vi "Select_Filename_List.vi"(4 "No dialogs":bool, 5 "File Type":string, 6 "Search String":string, 7 "At Dialog Prompt Post Process":T1, 8 "Previous Choice":path) -> (0 "Current Results filenames":path[](array[path]), 1 "Selected files":path[](array[path]), 3 "Choosen path":path)   [LabVIEW 2021]
uses:
  Controls/File_Selector_Type.ctl
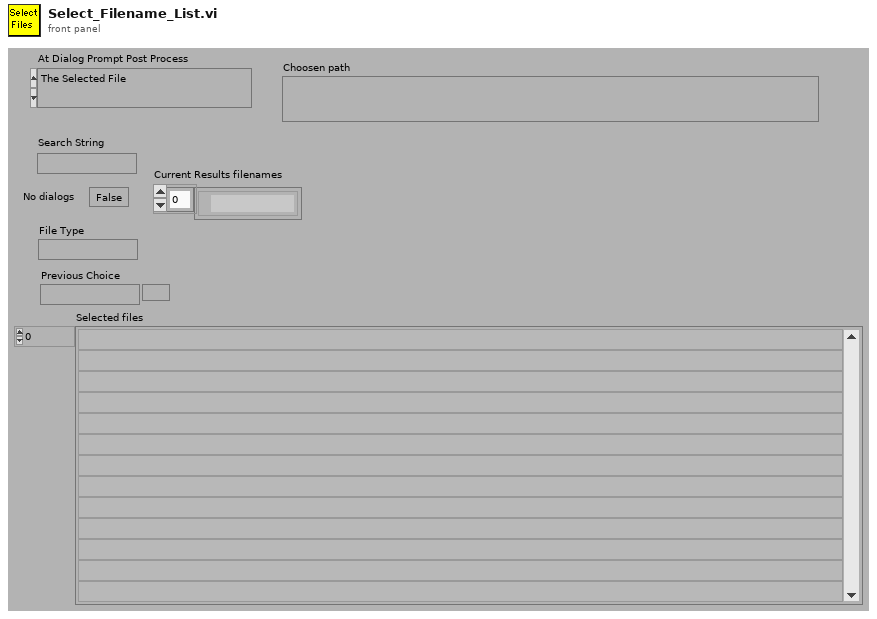
[diagram p1: front panel]
types:
  T1 = typedef "File_Selector_Type.ctl" = enum16{"The Selected File", "The Selected Folder", "Files containing the search string in the selected folder", "All files listed in selected file"}
  T2 = enum32{"existing file", "new file", "new or existing file", "existing dir", "new dir", "new or existing dir", "existing file (use LLBs)", "new file (use LLBs)", "new or existing file (use LLBs)", "new or existing file or directory (use LLBs)"}
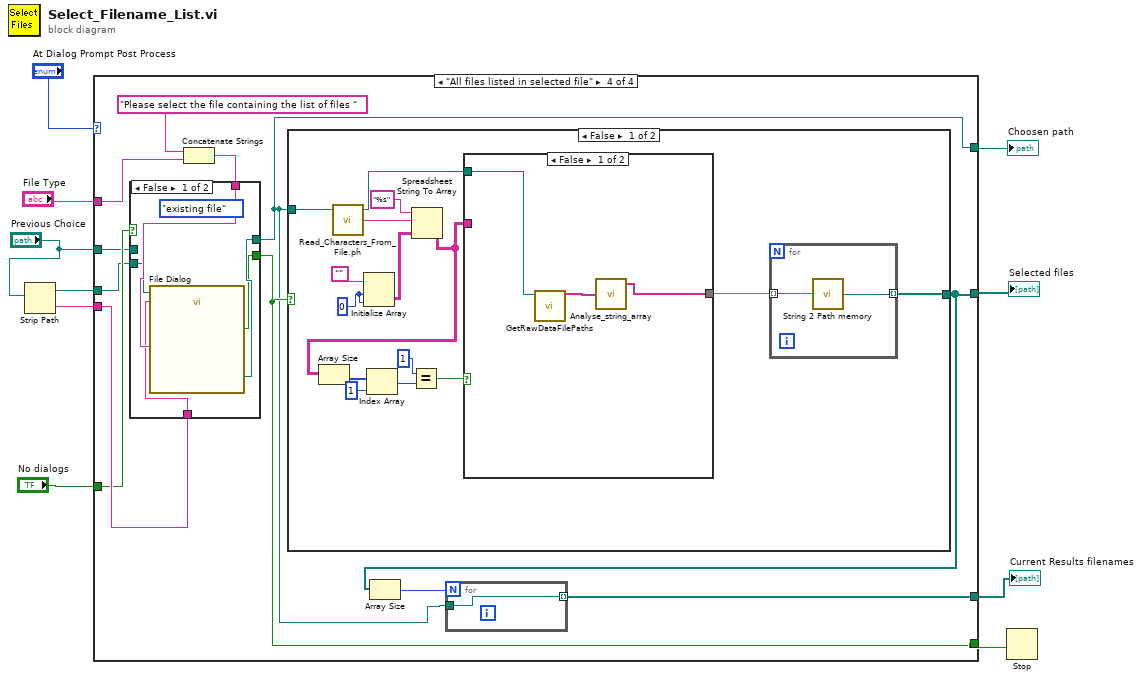
[diagram p0: block diagram]
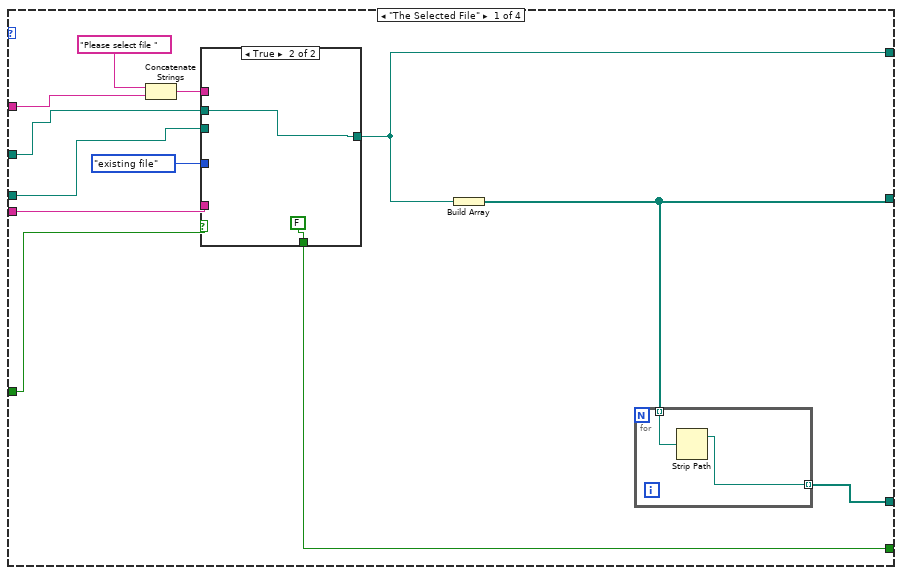
[diagram p2: hidden frame]
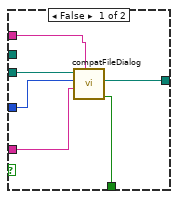
[diagram p3: hidden frame]
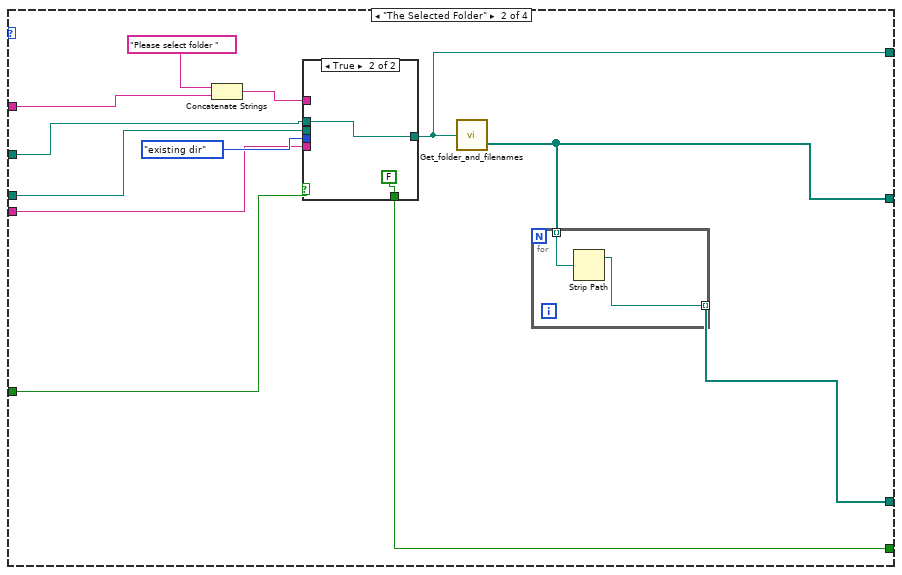
[diagram p4: hidden frame]
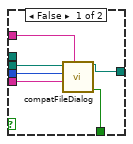
[diagram p5: hidden frame]
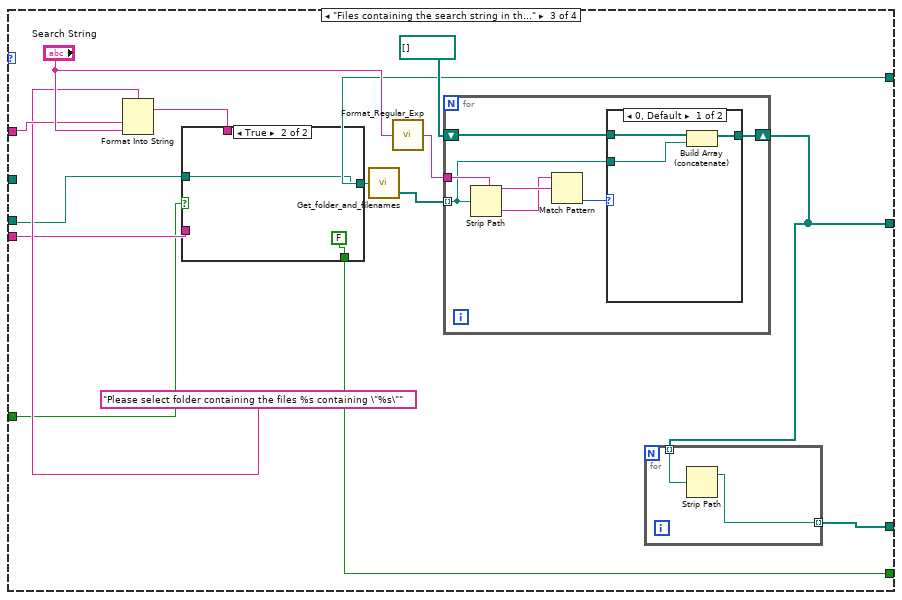
[diagram p6: hidden frame]
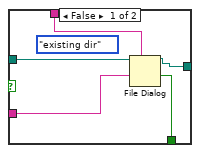
[diagram p7: hidden frame]
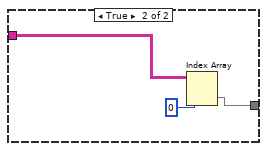
[diagram p9: hidden frame]
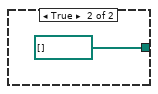
[diagram p10: hidden frame]
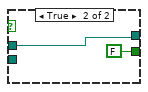
[diagram p11: hidden frame]
diagram:
  n1 = Strip Path(path="Previous Choice") -> (stripped path=w6:path, name=w5:string)
  n2 = case shown="\"All files listed in selected file\"" "At Dialog Prompt Post Process" {
    tunnel: [w13 w35 w55 w92] -> w7
    tunnel: "File Type" -> [w21 w42 w62 w98]
    tunnel: [w18 w43 w63 w93] -> w8
    tunnel: w6 -> [w17 w39 w60 w94]
    tunnel: w5 -> [w16 w38 w59 w96]
    tunnel: [w14 w37 w58 w89] -> w4
    tunnel: "No dialogs" -> [w15 w36 w57 w95]
    tunnel: [w12 w34 w56 w90] -> w2
    tunnel: "Previous Choice" -> [w11 w33 _ w88]
    frame "The Selected File" {
      n3 = Concatenate Strings("Please select file " ("prompt"), w21) -> (w19:string)
      n4 = case shown="True" w15 {
        tunnel: T2."existing file" ("select mode (2)") -> [w30 _]
        tunnel: w19 -> [w29 _]
        tunnel: [w28 FALSE ("cancelled")] -> w18
        tunnel: w17 -> [w27 _]
        tunnel: w16 -> [w26 _]
        tunnel: [w25 w31] -> w14
        tunnel: w11 -> [_ w31]
        frame False {
          n5 = call <vilib>:"compatFileDialog.vi"("prompt"=w29, "default name"=w26, "select mode (2)"=w30, "start path"=w27) -> ("cancelled"=w28:bool, "path"=w25:path)  [unwired: 3 in, 3 out]
        }
        frame True {
        }
      }
      n6 = Build Array(w14) -> (w13:path[])
      n7 = for {
        tunnel: w13 -> [w24] mode=indexing
        tunnel: [w23] -> w12 mode=indexing
        n8 = Strip Path(path=w24) -> (stripped path=w23:path)  [unwired: 1 out]
      }
    }
    frame "The Selected Folder" {
      n9 = Concatenate Strings("Please select folder " ("prompt"), w42) -> (w40:string)
      n10 = case shown="True" w36 {
        tunnel: T2."existing dir" ("select mode (2)") -> [w52 _]
        tunnel: [w51 FALSE ("cancelled")] -> w43
        tunnel: w40 -> [w50 _]
        tunnel: w39 -> [w49 _]
        tunnel: w38 -> [w48 _]
        tunnel: [w47 w53] -> w37
        tunnel: w33 -> [_ w53]
        frame False {
          n11 = call <vilib>:"compatFileDialog.vi"("prompt"=w50, "default name"=w48, "select mode (2)"=w52, "start path"=w49) -> ("cancelled"=w51:bool, "path"=w47:path)  [unwired: 3 in, 3 out]
        }
        frame True {
        }
      }
      n12 = call "Get_folder_and_filenames.vi"("file path (dialog if empty)"=w37) -> ("Files"=w35:path[])  [unwired: 1 out]
      n13 = for {
        tunnel: w35 -> [w46] mode=indexing
        tunnel: [w45] -> w34 mode=indexing
        n14 = Strip Path(path=w46) -> (stripped path=w45:path)  [unwired: 1 out]
      }
    }
    frame "Files containing the search string in the selected folder" {
      n15 = Format Into String(format string="Please select folder containing the files %s containing \"%s\"" ("prompt"), w62, "Search String") -> (resulting string=w68:string)  [unwired: 2 in, 1 out]
      n16 = case shown="True" w57 {
        tunnel: w68 -> [w75 _]
        tunnel: [w74 FALSE ("cancelled")] -> w63
        tunnel: w60 -> [w73 w77]
        tunnel: w59 -> [w72 _]
        tunnel: [w71 w77] -> w58
        frame False {
          (unwired) T2."existing dir" ("select mode (2)")
          n17 = File Dialog(7:w75, 9:w72, 11:w73) -> (1:w74:bool, 3:w71:path)  [unwired: 1 in, 5 out]
        }
        frame True {
        }
      }
      n18 = call "Get_folder_and_filenames.vi"("file path (dialog if empty)"=w58) -> ("Files"=w67:path[])  [unwired: 1 out]
      n19 = call "Format_Regular_Exp.vi"("Regular expression"="Search String") -> ("Case Insensitive for html"=w64:string)
      n20 = for {
        shift-right: [w78] -> w55
        shift-left: path[] [] -> [w80]
        tunnel: w64 -> [w83]
        tunnel: w67 -> [w79] mode=indexing
        n21 = Strip Path(path=w79) -> (name=w82:string)  [unwired: 1 out]
        n22 = Match Pattern(string=w82, regular expression=w83) -> (offset past match=w81:i32)  [unwired: 4 out]
        n23 = case shown="0, Default" w81 {
          tunnel: w80 -> [w86 w87]
          tunnel: w79 -> [w85 _]
          tunnel: [w84 w87] -> w78
          frame 0, Default {
            n24 = Build Array (concatenate)(w86, w85) -> (w84:path[])
          }
          frame -1 {
          }
        }
      }
      n25 = for {
        tunnel: w55 -> [w70] mode=indexing
        tunnel: [w69] -> w56 mode=indexing
        n26 = Strip Path(path=w70) -> (stripped path=w69:path)  [unwired: 1 out]
      }
    }
    frame "All files listed in selected file" {
      n27 = Concatenate Strings("Please select the file containing the list of files " ("prompt"), w98) -> (w97:string)
      n28 = case shown="False" w95 {
        tunnel: [w125 FALSE ("cancelled")] -> w93
        tunnel: w97 -> [w129 _]
        tunnel: w94 -> [w127 _]
        tunnel: w96 -> [w128 _]
        tunnel: [w126 w130] -> w89
        tunnel: w88 -> [_ w130]
        frame False {
          (unwired) T2."existing file" ("select mode (2)")
          n29 = call "File Dialog"("start path"=w127, "prompt"=w129, "default name"=w128) -> ("selected path"=w126:path, "cancelled"=w125:bool)  [unwired: 9 in, 2 out]
        }
        frame True {
        }
      }
      n30 = case shown="False" w93 {
        tunnel: w89 -> [w104 _]
        tunnel: [w102 path[] []] -> w92
        frame False {
          w111 = 0 ("Dimension Size")
          n31 = call "Read_Characters_From_File.ph.vi"("file path (dialog if empty)"=w104) -> ("new file path (NotAPath if cancelled)"=w101:path, "character string"=w115:string)  [unwired: 1 in, 6 out]
          n32 = Initialize Array("", w111, w111) -> (w113:string[][])
          n33 = Spreadsheet String To Array(format string="%s", spreadsheet string=w115, array type (2D Dbl)=w113) -> (array=w110:string[][])  [unwired: 1 out]
          n34 = Array Size(array=w110) -> (size(s)=w109:i32[])
          n35 = Index Array(array=w109, index=1) -> (element=w107:i32)
          n36 = Equal?(x=1, y=w107) -> (x = y?=w105:bool)
          n37 = case shown="False" w105 {
            tunnel: w110 -> [_ w123]
            tunnel: w101 -> [w120 _]
            tunnel: [w118 w121] -> w103
            frame False {
              n38 = call "GetRawDataFilePaths.vi"("Results file or Folder"=w120) -> ("RawDataFilePaths"=w119:string[])  [unwired: 10 in]
              n39 = call "Analyse_string_array.vi"("String array"=w119) -> ("Unique strings"=w118:string[])  [unwired: 1 in, 1 out]
            }
            frame True {
              n40 = Index Array(array=w123, index (col)=0 ("disabled index (col)")) -> (element=w121:string[])  [unwired: 1 in]
            }
          }
          n41 = for {
            tunnel: w103 -> [w117] mode=indexing
            tunnel: [w116] -> w102 mode=indexing
            n42 = call "String 2 Path memory.vi"("Input String"=w117) -> ("path"=w116:path)  [unwired: 1 in]
          }
        }
        frame True {
        }
      }
      n43 = Array Size(array=w92) -> (size(s)=w91:i32)
      n44 = for {
        N: w91 -> [_]
        tunnel: [w100] -> w90 mode=indexing
        tunnel: w89 -> [w100]
      }
    }
  }
  "Selected files" <- w7
  "Choosen path" <- w4
  "Current Results filenames" <- w2
  n45 = Stop(stop? (T)=w8) -> ()
